vi "Linear K Data Demo.vi"() -> ()   [LabVIEW 2012]
uses:
  LabVIEW/user.lib/SpectralRadar.llb/Calibration Selection.ctl
  LabVIEW/user.lib/SpectralRadar.llb/Data 2D Export Format Selection.ctl
  LabVIEW/user.lib/SpectralRadar.llb/set Spectrum Output.vi
  LabVIEW/user.lib/SpectralRadar.llb/set Complex Scan Output.vi
  LabVIEW/user.lib/SpectralRadar.llb/display Data 1D.vi
  LabVIEW/user.lib/SpectralRadar.llb/display Data 2D.vi
  LabVIEW/user.lib/SpectralRadar.llb/OCT Device.lvclass
  LabVIEW/user.lib/SpectralRadar.llb/Processing.lvclass
  LabVIEW/user.lib/SpectralRadar.llb/Raw Data.lvclass
  LabVIEW/user.lib/SpectralRadar.llb/Data.lvclass
  LabVIEW/user.lib/SpectralRadar.llb/Complex Data.lvclass
panel:
  out "Raw Spectrum":dbl[](graph)
  out "Linear K Spectrum":dbl[](graph)
  in  "Save":bool
  in  "Apo":bool
  in  "stop":bool
  out "Spectral Data":dbl[][](graph)
  in  "AScans / BScan":i32=512
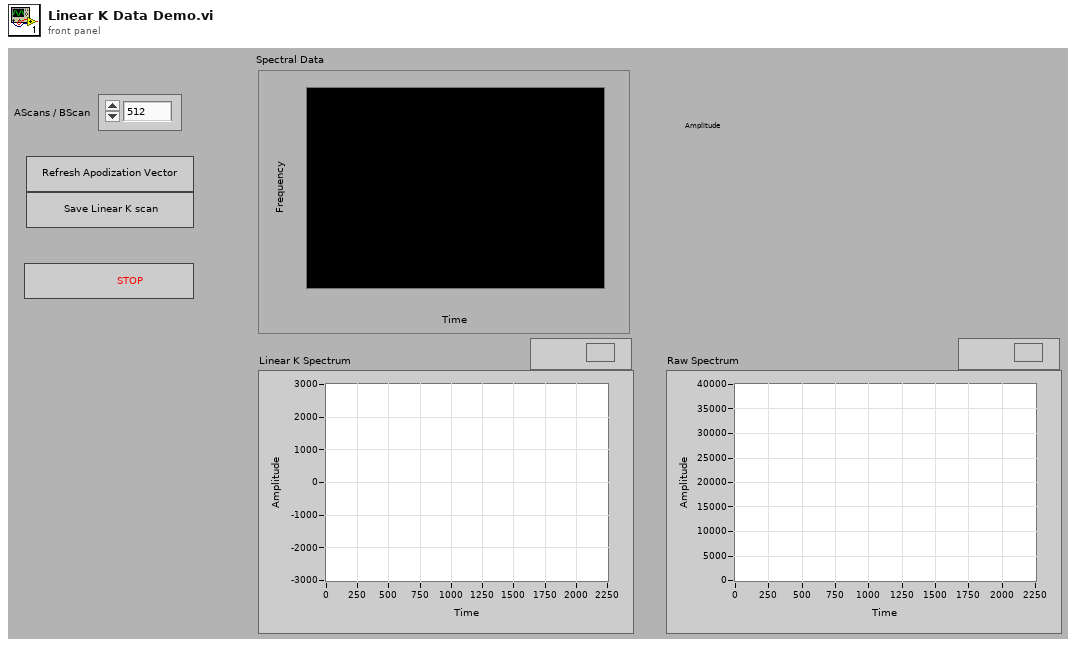
[diagram p1: front panel]
types:
  T1 = typedef "Data.lvclass/Data 2D Export Format Selection.ctl" = enum16{"SRM (Spectral Radar Metafile)", "RAW", "TXT", "CSV", "TXT Table"}
  T2 = typedef "Processing.lvclass/Calibration Selection.ctl" = enum16{"Offset Errors", "Apodization Spectrum", "Apodization Vector", "Dispersion", "Chirp", "Extended Adjust", "Fixed Pattern"}
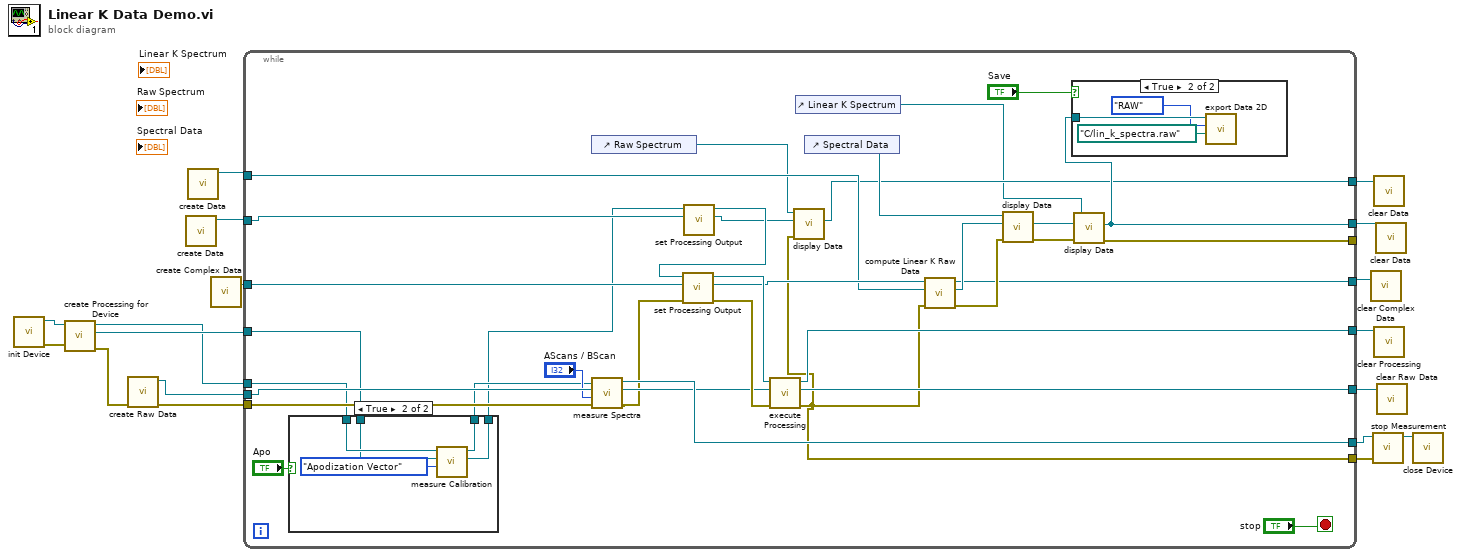
[diagram p0: block diagram]
diagram:
  n1 = call "init Device.vi"() -> ("error out"=w18:errorcluster, "OCTDevice"=w13:refnum<class "OCT Device.lvclass">)  [unwired: 6 in]
  n2 = call "create Processing for Device.vi"("error in (no error)"=w18, "OCTDevice"=w13) -> ("error out"=w7:errorcluster, "Processing"=w15:refnum<class "Processing.lvclass">, "OCTDevice"=w8:refnum<class "OCT Device.lvclass">)  [unwired: 3 in]
  n3 = call "create Raw Data.vi"("error in (no error)"=w7) -> ("error out"=w16:errorcluster, "Raw Data"=w17:refnum<class "Raw Data.lvclass">)  [unwired: 5 in]
  n4 = call "create Data.vi"() -> ("Data"=w5:refnum<class "Data.lvclass">)  [unwired: 6 in, 1 out]
  n5 = call "create Data.vi"() -> ("Data"=w4:refnum<class "Data.lvclass">)  [unwired: 6 in, 1 out]
  n6 = call "create Complex Data.vi"() -> ("Complex Data"=w10:refnum<class "Complex Data.lvclass">)  [unwired: 2 in, 1 out]
  n7 = while {
    tunnel: w17 -> [w43]
    tunnel: w8 -> [w37]
    tunnel: w16 -> [w42]
    tunnel: w15 -> [w35]
    tunnel: w10 -> [w53]
    tunnel: [w50] -> w14
    tunnel: [w47] -> w1
    tunnel: [w28] -> w3
    tunnel: [w41] -> w12
    tunnel: w4 -> [w45]
    tunnel: [w21] -> w9
    tunnel: [w30] -> _
    tunnel: [w29] -> w6
    tunnel: w5 -> [w26]
    tunnel: [w22] -> w2
    stop <- "stop" stop-if-true
    n8 = case shown="True" "Apo" {
      tunnel: w37 -> [w57 w63]
      tunnel: [w57 w62] -> w36
      tunnel: w35 -> [w58 w61]
      tunnel: [w58 w60] -> w25
      frame False {
      }
      frame True {
        n9 = call "measure Calibration.vi"("Calibration Data"=Calibration_Selection."Apodization Vector", "Processing"=w61, "OCTDevice"=w63) -> ("Processing"=w60:refnum<class "Processing.lvclass">, "OCTDevice"=w62:refnum<class "OCT Device.lvclass">)  [unwired: 3 in, 1 out]
      }
    }
    n10 = control-ref of="Raw Spectrum"() -> (w19:refnum<vi>)
    n11 = call "measure Spectra.vi"("error in (no error)"=w42, "NumberOfSpectra"="AScans / BScan", "Raw Data"=w43, "OCTDevice"=w36) -> ("error out"=w39:errorcluster, "Raw Data"=w40:refnum<class "Raw Data.lvclass">, "OCTDevice"=w41:refnum<class "OCT Device.lvclass">)  [unwired: 2 in]
    n12 = call-poly "set Processing Output.vi"("Data"=w26, "Processing"=w25) -> ("Data"=w23:refnum<class "Data.lvclass">, "Processing"=w24:refnum<class "Processing.lvclass">)  [unwired: 3 in, 1 out]
    n13 = call-poly "set Processing Output.vi"("error in (no error)"=w39, "Complex Data in"=w53, "Processing"=w24) -> ("error out"=w52:errorcluster, "Complex Data out"=w46:refnum<class "Complex Data.lvclass">, "Processing"=w48:refnum<class "Processing.lvclass">)  [unwired: 2 in]
    n14 = call "execute Processing.vi"("error in (no error)"=w52, "Raw Data"=w40, "Processing"=w48) -> ("error out"=w21:errorcluster, "Raw Data"=w50:refnum<class "Raw Data.lvclass">, "Processing"=w47:refnum<class "Processing.lvclass">)  [unwired: 2 in]
    n15 = call-poly "display Data.vi"("error in (no error)"=w21, "Data in"=w23, "WFGraph Refnum"=w19) -> ("Data out"=w22:refnum<class "Data.lvclass">)  [unwired: 2 in, 2 out]
    n16 = control-ref of="Linear K Spectrum"() -> (w20:refnum<vi>)
    n17 = control-ref of="Spectral Data"() -> (w51:refnum<vi>)
    n18 = call "compute Linear K Raw Data.vi"("error in (no error)"=w21, "Data"=w45, "Complex Data in"=w46) -> ("error out"=w33:errorcluster, "Data out"=w44:refnum<class "Data.lvclass">, "Complex Data out"=w29:refnum<class "Complex Data.lvclass">)  [unwired: 2 in]
    n19 = call-poly "display Data.vi"("error in (no error)"=w33, "Data in"=w44, "IntGraph Refnum"=w51) -> ("error out"=w31:errorcluster, "Data out"=w32:refnum<class "Data.lvclass">)  [unwired: 2 in, 1 out]
    n20 = call-poly "display Data.vi"("error in (no error)"=w31, "Data in"=w32, "WFGraph Refnum"=w20) -> ("error out"=w30:errorcluster, "Data out"=w28:refnum<class "Data.lvclass">)  [unwired: 2 in, 1 out]
    n21 = case shown="True" "Save" {
      tunnel: w28 -> [_ w56]
      frame False {
      }
      frame True {
        n22 = call "export Data 2D.vi"("Export File"=path "C:/lin_k_spectra.raw", "Data 2D Export Format Selection"=Data_2D_Export_Format_Selection."RAW", "Data in"=w56) -> ()  [unwired: 3 in, 2 out]
      }
    }
  }
  n23 = call "clear Complex Data.vi"("Complex Data"=w6) -> ()  [unwired: 6 in, 1 out]
  n24 = call "stop Measurement.vi"("error in (no error)"=w9, "OCTDevice"=w12) -> ("OCTDevice"=w11:refnum<class "OCT Device.lvclass">)  [unwired: 4 in, 1 out]
  n25 = call "clear Data.vi"("Data"=w2) -> ()  [unwired: 6 in, 1 out]
  n26 = call "clear Processing.vi"("Processing"=w1) -> ()  [unwired: 6 in, 1 out]
  n27 = call "clear Data.vi"("Data"=w3) -> ()  [unwired: 6 in, 1 out]
  n28 = call "clear Raw Data.vi"("Raw Data"=w14) -> ()  [unwired: 6 in, 1 out]
  n29 = call "close Device.vi"("OCTDevice"=w11) -> ()  [unwired: 6 in, 1 out]
